vi "Nan_inf_removing.vi"(3 "All?":bool, 4 "II channel seq IN in":cluster{"BG":sgl[], "Ie":sgl[], "I0":sgl[]}[](array[cluster]), 5 "I channel seq IN in":cluster{"BG":sgl[], "Ie":sgl[], "I0":sgl[]}[](array[cluster])) -> (0 "I channel out":cluster{"BG":sgl[], "Ie":sgl[], "I0":sgl[]}[](array[cluster]), 1 "II channel out":cluster{"BG":sgl[], "Ie":sgl[], "I0":sgl[]}[](array[cluster]))   [LabVIEW 2020, in "Detector.lvclass"]
uses:
  Detector.lvclass
  dependecies/globalVarII.vi
  <userlib>/_OpenG.lib/array/array.llb/Search 1D Array (SGL)__ogtk.vi
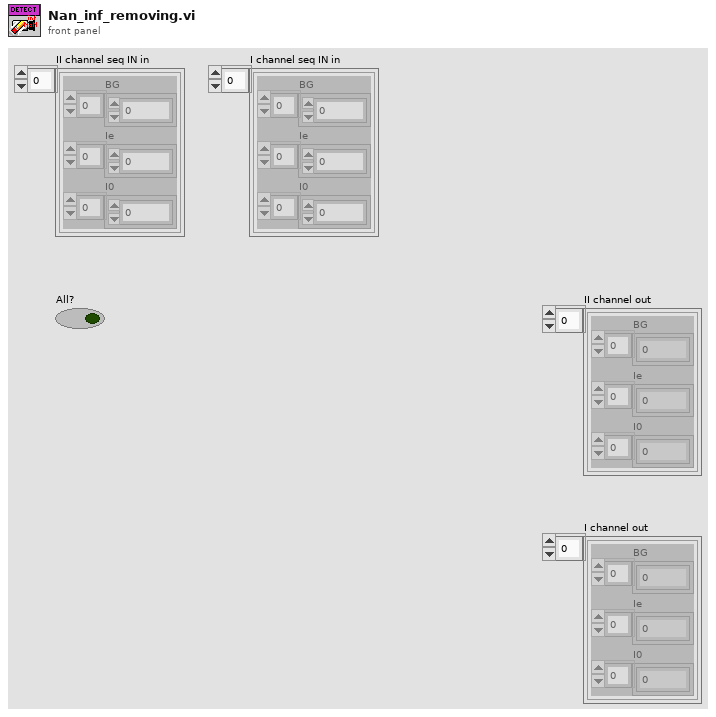
[diagram p1: front panel]
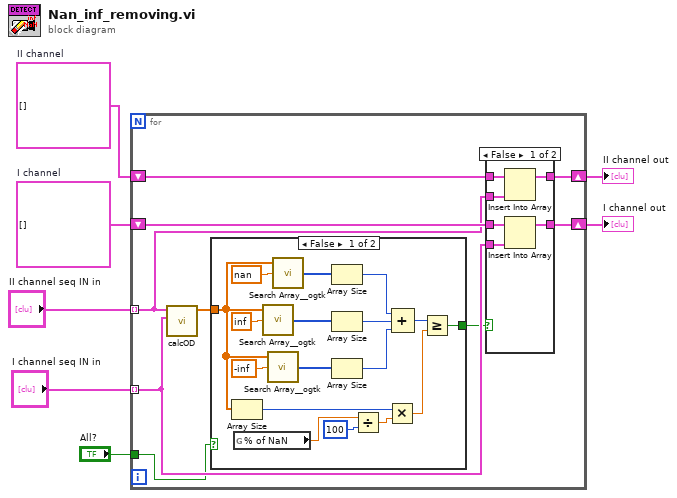
[diagram p0: block diagram]
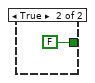
[diagram p2: hidden frame]
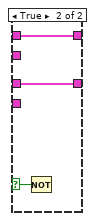
[diagram p3: hidden frame]
diagram:
  w6 = cluster{"BG":sgl[], "Ie":sgl[], "I0":sgl[]}[] []  # II channel
  w5 = cluster{"BG":sgl[], "Ie":sgl[], "I0":sgl[]}[] []  # I channel
  n1 = for {
    tunnel: "I channel seq IN in" -> [w12] mode=indexing
    tunnel: "II channel seq IN in" -> [w13] mode=indexing
    shift-right: [w10] -> w4
    shift-left: w5 -> [w15]
    shift-right: [w11] -> w3
    shift-left: w6 -> [w14]
    tunnel: "All?" -> [w8]
    n2 = call "calcOD.vi"("channel I"=w12, "channel 2"=w13) -> ("OD"=w16:sgl[])  [unwired: 3 in, 6 out]
    n3 = case shown="False" w8 {
      tunnel: w16 -> [w31 _]
      tunnel: [w17 FALSE] -> w9
      frame False {
        n4 = Array Size(array=w31) -> (size(s)=w30:i32)
        n5 = global read "globalVarII.vi" "% of NaN"() -> (w24:sgl)
        n6 = call-poly <userlib>:"Search Array__ogtk.vi"("Array"=w31, "Element Data"=sgl inf) -> ("Indices of Elements"=w29:i32[])  [unwired: 7 in]
        n7 = call-poly <userlib>:"Search Array__ogtk.vi"("Array"=w31, "Element Data"=sgl -inf) -> ("Indices of Elements"=w28:i32[])  [unwired: 7 in]
        n8 = call-poly <userlib>:"Search Array__ogtk.vi"("Array"=w31, "Element Data"=sgl nan) -> ("Indices of Elements"=w32:i32[])  [unwired: 7 in]
        n9 = Array Size(array=w32) -> (size(s)=w22:i32)
        n10 = Array Size(array=w29) -> (size(s)=w21:i32)
        n11 = Array Size(array=w28) -> (size(s)=w20:i32)
        n12 = Divide(x=w24, y=100) -> (x/y=w25:sgl)
        n13 = Multiply(x=w30, y=w25) -> (x*y=w18:sgl)
        n14 = Compound Arithmetic op=ADD(w22, w21, w20) -> (w19:i32)
        n15 = Greater Or Equal?(x=w19, y=w18) -> (x >= y?=w17:bool)
      }
      frame True {
      }
    }
    n16 = case shown="False" w9 {
      selector: w9 -> [_ w41]
      tunnel: w15 -> [w40 w42]
      tunnel: w12 -> [w39 _]
      tunnel: [w38 w42] -> w10
      tunnel: [w37 w43] -> w11
      tunnel: w14 -> [w36 w43]
      tunnel: w13 -> [w35 _]
      frame False {
        n17 = Insert Into Array(array=w36, new element=w35) -> (w37:cluster{"BG":sgl[], "Ie":sgl[], "I0":sgl[]}[])  [unwired: 1 in]
        n18 = Insert Into Array(array=w40, new element=w39) -> (w38:cluster{"BG":sgl[], "Ie":sgl[], "I0":sgl[]}[])  [unwired: 1 in]
      }
      frame True {
        n19 = Not(x=w41) -> ()  [unwired: 1 out]
      }
    }
  }
  "I channel out" <- w4
  "II channel out" <- w3
